vi "SetPIDVelocityGains.vi"(10 "Velocity PID gains":T1={"proportional gain (Kc)"=1.0, "integral time (Ti, min)"=0.01, "derivative time (Td, min)"=0.0} {"derivative time (Td, min)" format="%.3f"; "integral time (Ti, min)" format="%.3f"; "proportional gain (Kc)" format="%.3f"}, 11 "DriveBase.lvclass":refnum<class "DriveBase.lvclass">) -> (3 "DriveBase.lvclass 2":refnum<class "DriveBase.lvclass">)   [LabVIEW 2016, in "DriveBase.lvclass"]
uses:
  DriveBase.lvclass
  DriveBase.lvclass/DriveBase.ctl
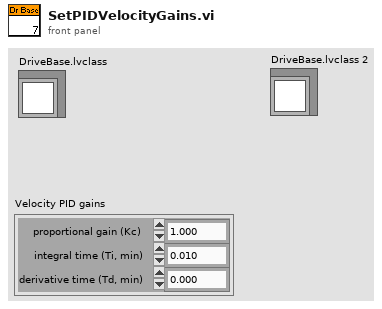
[diagram p1: front panel]
types:
  T1 = cluster{"proportional gain (Kc)":dbl, "integral time (Ti, min)":dbl, "derivative time (Td, min)":dbl}
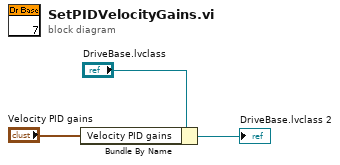
[diagram p0: block diagram]
diagram:
  n1 = Bundle By Name(cluster="DriveBase.lvclass", "Velocity PID gains"="Velocity PID gains") -> (→"DriveBase.lvclass 2":refnum<class "DriveBase.lvclass">)
